vi "dispose configuration.vi"(8 "error in":errorcluster, 11 "lvlibretls configurable context in":refnum<class "lvlibretls configurable context.lvclass">) -> (0 "error out":errorcluster)   [LabVIEW 2016, in "lvlibretls configurable context.lvclass"]
uses:
  lvlibretls configurable context.lvclass
  lvlibretls configurable context.lvclass/lvlibretls configurable context.ctl
  lv tls dll.lvlib
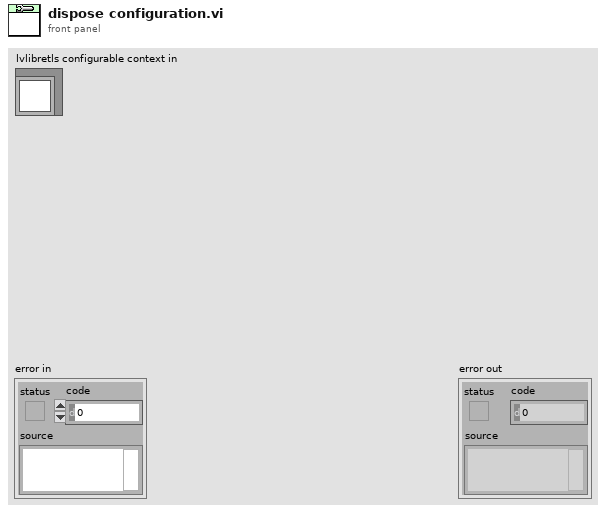
[diagram p1: front panel]
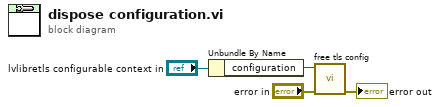
[diagram p0: block diagram]
diagram:
  n1 = Unbundle By Name("lvlibretls configurable context in") -> ("configuration"=w1:u64)
  n2 = call "free tls config.vi"("error in"="error in", "config"=w1) -> ("error out"=→"error out":errorcluster)  [unwired: 9 in]
